vi "SaccadeAnalyser - Auto Select Channels.vi"(11 "plane":T1=enum."Yaw" caption="Impulse Plane") -> (1 "Position Response Channel":u16(ring)=7 items=["Hz Position-in-Head", "Hz Velocity-in-Head", "Hy Position-in-Head", "Hy Velocity-in-Head", "Hx Position-in-Head", "Hx Velocity-in-Head", "Hl Velocity-in-Head", "Hr Velocity-in-Head", "Lx Position-in-Head", "Ly Position-in-Head", "Lz Position-in-Head", "Lx Velocity-in-Head", "Ly Velocity-in-Head", "Lz Velocity-in-Head", "Ll Velocity-in-Head", "Lr Velocity-in-Head", "Rx Position-in-Head", "Ry Position-in-Head", "Rz Position-in-Head", "Rx Velocity-in-Head", "Ry Velocity-in-Head", "Rz Velocity-in-Head", "Rl Velocity-in-Head", "Rr Velocity-in-Head", "Target on/off", "aux input 1", "aux input 2", " ", "", "", "", "Target Hor", "Target Ver", ""], 2 "Velocity Response Channel":u16(ring)=7 items=["Hz Position-in-Head", "Hz Velocity-in-Head", "Hy Position-in-Head", "Hy Velocity-in-Head", "Hx Position-in-Head", "Hx Velocity-in-Head", "Hl Velocity-in-Head", "Hr Velocity-in-Head", "Lx Position-in-Head", "Ly Position-in-Head", "Lz Position-in-Head", "Lx Velocity-in-Head", "Ly Velocity-in-Head", "Lz Velocity-in-Head", "Ll Velocity-in-Head", "Lr Velocity-in-Head", "Rx Position-in-Head", "Ry Position-in-Head", "Rz Position-in-Head", "Rx Velocity-in-Head", "Ry Velocity-in-Head", "Rz Velocity-in-Head", "Rl Velocity-in-Head", "Rr Velocity-in-Head", "Target on/off", "aux input 1", "aux input 2", " ", "", "", "", "Target Hor", "Target Ver", ""], 3 "Stimulus Channel":u16(ring)=7 items=["Hz Position-in-Head", "Hz Velocity-in-Head", "Hy Position-in-Head", "Hy Velocity-in-Head", "Hx Position-in-Head", "Hx Velocity-in-Head", "Hl Velocity-in-Head", "Hr Velocity-in-Head", "Lx Position-in-Head", "Ly Position-in-Head", "Lz Position-in-Head", "Lx Velocity-in-Head", "Ly Velocity-in-Head", "Lz Velocity-in-Head", "Ll Velocity-in-Head", "Lr Velocity-in-Head", "Rx Position-in-Head", "Ry Position-in-Head", "Rz Position-in-Head", "Rx Velocity-in-Head", "Ry Velocity-in-Head", "Rz Velocity-in-Head", "Rl Velocity-in-Head", "Rr Velocity-in-Head", "Target on/off", "aux input 1", "aux input 2", " ", "", "", "", "Target Hor", "Target Ver", ""])   [LabVIEW 2016]
uses:
  Type Definitions/Saccade Analyser Impulse Plane.ctl
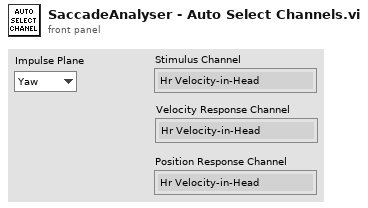
[diagram p1: front panel]
types:
  T1 = typedef "Saccade Analyser Impulse Plane.ctl" = enum16{"Other", "Yaw", "Pitch", "Roll", "LARP", "RALP"}
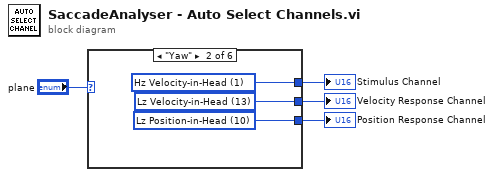
[diagram p0: block diagram]
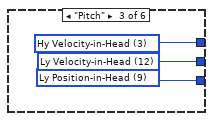
[diagram p3: hidden frame]
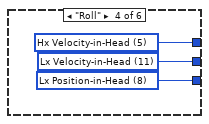
[diagram p4: hidden frame]
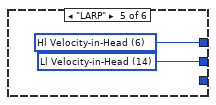
[diagram p5: hidden frame]
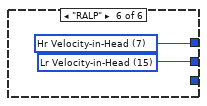
[diagram p6: hidden frame]
diagram:
  n1 = case shown="\"Yaw\"" "plane" {
    tunnel: [_ w7 w10 w13 w15 w17] -> w3
    tunnel: [_ w6 w9 w12 w14 w16] -> w2
    tunnel: [_ w5 w8 w11 _ _] -> w1
    frame "Other", Default {
      # "No default selections for these planes."
    }
    frame "Yaw" {
      w5 = u16 10 items=["Hz Position-in-Head", "Hz Velocity-in-Head", "Hy Position-in-Head", "Hy Velocity-in-Head", "Hx Position-in-Head", "Hx Velocity-in-Head", "Hl Velocity-in-Head", "Hr Velocity-in-Head", "Lx Position-in-Head", "Ly Position-in-Head", "Lz Position-in-Head", "Lx Velocity-in-Head", "Ly Velocity-in-Head", "Lz Velocity-in-Head", "Ll Velocity-in-Head", "Lr Velocity-in-Head", "Rx Position-in-Head", "Ry Position-in-Head", "Rz Position-in-Head", "Rx Velocity-in-Head", "Ry Velocity-in-Head", "Rz Velocity-in-Head", "Rl Velocity-in-Head", "Rr Velocity-in-Head", "Target on/off", "aux input 1", "aux input 2", " ", "", "", "", "Target Hor", "Target Ver", ""] ("ring_response channel")
      w6 = u16 13 items=["Hz Position-in-Head", "Hz Velocity-in-Head", "Hy Position-in-Head", "Hy Velocity-in-Head", "Hx Position-in-Head", "Hx Velocity-in-Head", "Hl Velocity-in-Head", "Hr Velocity-in-Head", "Lx Position-in-Head", "Ly Position-in-Head", "Lz Position-in-Head", "Lx Velocity-in-Head", "Ly Velocity-in-Head", "Lz Velocity-in-Head", "Ll Velocity-in-Head", "Lr Velocity-in-Head", "Rx Position-in-Head", "Ry Position-in-Head", "Rz Position-in-Head", "Rx Velocity-in-Head", "Ry Velocity-in-Head", "Rz Velocity-in-Head", "Rl Velocity-in-Head", "Rr Velocity-in-Head", "Target on/off", "aux input 1", "aux input 2", " ", "", "", "", "Target Hor", "Target Ver", ""] ("ring_response channel")
      w7 = u16 1 items=["Hz Position-in-Head", "Hz Velocity-in-Head", "Hy Position-in-Head", "Hy Velocity-in-Head", "Hx Position-in-Head", "Hx Velocity-in-Head", "Hl Velocity-in-Head", "Hr Velocity-in-Head", "Lx Position-in-Head", "Ly Position-in-Head", "Lz Position-in-Head", "Lx Velocity-in-Head", "Ly Velocity-in-Head", "Lz Velocity-in-Head", "Ll Velocity-in-Head", "Lr Velocity-in-Head", "Rx Position-in-Head", "Ry Position-in-Head", "Rz Position-in-Head", "Rx Velocity-in-Head", "Ry Velocity-in-Head", "Rz Velocity-in-Head", "Rl Velocity-in-Head", "Rr Velocity-in-Head", "Target on/off", "aux input 1", "aux input 2", " ", "", "", "", "Target Hor", "Target Ver", ""] ("ring_stimulus channel")
    }
    frame "Pitch" {
      w8 = u16 9 items=["Hz Position-in-Head", "Hz Velocity-in-Head", "Hy Position-in-Head", "Hy Velocity-in-Head", "Hx Position-in-Head", "Hx Velocity-in-Head", "Hl Velocity-in-Head", "Hr Velocity-in-Head", "Lx Position-in-Head", "Ly Position-in-Head", "Lz Position-in-Head", "Lx Velocity-in-Head", "Ly Velocity-in-Head", "Lz Velocity-in-Head", "Ll Velocity-in-Head", "Lr Velocity-in-Head", "Rx Position-in-Head", "Ry Position-in-Head", "Rz Position-in-Head", "Rx Velocity-in-Head", "Ry Velocity-in-Head", "Rz Velocity-in-Head", "Rl Velocity-in-Head", "Rr Velocity-in-Head", "Target on/off", "aux input 1", "aux input 2", " ", "", "", "", "Target Hor", "Target Ver", ""] ("ring_response channel")
      w9 = u16 12 items=["Hz Position-in-Head", "Hz Velocity-in-Head", "Hy Position-in-Head", "Hy Velocity-in-Head", "Hx Position-in-Head", "Hx Velocity-in-Head", "Hl Velocity-in-Head", "Hr Velocity-in-Head", "Lx Position-in-Head", "Ly Position-in-Head", "Lz Position-in-Head", "Lx Velocity-in-Head", "Ly Velocity-in-Head", "Lz Velocity-in-Head", "Ll Velocity-in-Head", "Lr Velocity-in-Head", "Rx Position-in-Head", "Ry Position-in-Head", "Rz Position-in-Head", "Rx Velocity-in-Head", "Ry Velocity-in-Head", "Rz Velocity-in-Head", "Rl Velocity-in-Head", "Rr Velocity-in-Head", "Target on/off", "aux input 1", "aux input 2", " ", "", "", "", "Target Hor", "Target Ver", ""] ("ring_response channel")
      w10 = u16 3 items=["Hz Position-in-Head", "Hz Velocity-in-Head", "Hy Position-in-Head", "Hy Velocity-in-Head", "Hx Position-in-Head", "Hx Velocity-in-Head", "Hl Velocity-in-Head", "Hr Velocity-in-Head", "Lx Position-in-Head", "Ly Position-in-Head", "Lz Position-in-Head", "Lx Velocity-in-Head", "Ly Velocity-in-Head", "Lz Velocity-in-Head", "Ll Velocity-in-Head", "Lr Velocity-in-Head", "Rx Position-in-Head", "Ry Position-in-Head", "Rz Position-in-Head", "Rx Velocity-in-Head", "Ry Velocity-in-Head", "Rz Velocity-in-Head", "Rl Velocity-in-Head", "Rr Velocity-in-Head", "Target on/off", "aux input 1", "aux input 2", " ", "", "", "", "Target Hor", "Target Ver", ""] ("ring_stimulus channel")
    }
    frame "Roll" {
      w11 = u16 8 items=["Hz Position-in-Head", "Hz Velocity-in-Head", "Hy Position-in-Head", "Hy Velocity-in-Head", "Hx Position-in-Head", "Hx Velocity-in-Head", "Hl Velocity-in-Head", "Hr Velocity-in-Head", "Lx Position-in-Head", "Ly Position-in-Head", "Lz Position-in-Head", "Lx Velocity-in-Head", "Ly Velocity-in-Head", "Lz Velocity-in-Head", "Ll Velocity-in-Head", "Lr Velocity-in-Head", "Rx Position-in-Head", "Ry Position-in-Head", "Rz Position-in-Head", "Rx Velocity-in-Head", "Ry Velocity-in-Head", "Rz Velocity-in-Head", "Rl Velocity-in-Head", "Rr Velocity-in-Head", "Target on/off", "aux input 1", "aux input 2", " ", "", "", "", "Target Hor", "Target Ver", ""] ("ring_response channel")
      w12 = u16 11 items=["Hz Position-in-Head", "Hz Velocity-in-Head", "Hy Position-in-Head", "Hy Velocity-in-Head", "Hx Position-in-Head", "Hx Velocity-in-Head", "Hl Velocity-in-Head", "Hr Velocity-in-Head", "Lx Position-in-Head", "Ly Position-in-Head", "Lz Position-in-Head", "Lx Velocity-in-Head", "Ly Velocity-in-Head", "Lz Velocity-in-Head", "Ll Velocity-in-Head", "Lr Velocity-in-Head", "Rx Position-in-Head", "Ry Position-in-Head", "Rz Position-in-Head", "Rx Velocity-in-Head", "Ry Velocity-in-Head", "Rz Velocity-in-Head", "Rl Velocity-in-Head", "Rr Velocity-in-Head", "Target on/off", "aux input 1", "aux input 2", " ", "", "", "", "Target Hor", "Target Ver", ""] ("ring_response channel")
      w13 = u16 5 items=["Hz Position-in-Head", "Hz Velocity-in-Head", "Hy Position-in-Head", "Hy Velocity-in-Head", "Hx Position-in-Head", "Hx Velocity-in-Head", "Hl Velocity-in-Head", "Hr Velocity-in-Head", "Lx Position-in-Head", "Ly Position-in-Head", "Lz Position-in-Head", "Lx Velocity-in-Head", "Ly Velocity-in-Head", "Lz Velocity-in-Head", "Ll Velocity-in-Head", "Lr Velocity-in-Head", "Rx Position-in-Head", "Ry Position-in-Head", "Rz Position-in-Head", "Rx Velocity-in-Head", "Ry Velocity-in-Head", "Rz Velocity-in-Head", "Rl Velocity-in-Head", "Rr Velocity-in-Head", "Target on/off", "aux input 1", "aux input 2", " ", "", "", "", "Target Hor", "Target Ver", ""] ("ring_stimulus channel")
    }
    frame "LARP" {
      w14 = u16 14 items=["Hz Position-in-Head", "Hz Velocity-in-Head", "Hy Position-in-Head", "Hy Velocity-in-Head", "Hx Position-in-Head", "Hx Velocity-in-Head", "Hl Velocity-in-Head", "Hr Velocity-in-Head", "Lx Position-in-Head", "Ly Position-in-Head", "Lz Position-in-Head", "Lx Velocity-in-Head", "Ly Velocity-in-Head", "Lz Velocity-in-Head", "Ll Velocity-in-Head", "Lr Velocity-in-Head", "Rx Position-in-Head", "Ry Position-in-Head", "Rz Position-in-Head", "Rx Velocity-in-Head", "Ry Velocity-in-Head", "Rz Velocity-in-Head", "Rl Velocity-in-Head", "Rr Velocity-in-Head", "Target on/off", "aux input 1", "aux input 2", " ", "", "", "", "Target Hor", "Target Ver", ""] ("ring_response channel")
      w15 = u16 6 items=["Hz Position-in-Head", "Hz Velocity-in-Head", "Hy Position-in-Head", "Hy Velocity-in-Head", "Hx Position-in-Head", "Hx Velocity-in-Head", "Hl Velocity-in-Head", "Hr Velocity-in-Head", "Lx Position-in-Head", "Ly Position-in-Head", "Lz Position-in-Head", "Lx Velocity-in-Head", "Ly Velocity-in-Head", "Lz Velocity-in-Head", "Ll Velocity-in-Head", "Lr Velocity-in-Head", "Rx Position-in-Head", "Ry Position-in-Head", "Rz Position-in-Head", "Rx Velocity-in-Head", "Ry Velocity-in-Head", "Rz Velocity-in-Head", "Rl Velocity-in-Head", "Rr Velocity-in-Head", "Target on/off", "aux input 1", "aux input 2", " ", "", "", "", "Target Hor", "Target Ver", ""] ("ring_stimulus channel")
    }
    frame "RALP" {
      w16 = u16 15 items=["Hz Position-in-Head", "Hz Velocity-in-Head", "Hy Position-in-Head", "Hy Velocity-in-Head", "Hx Position-in-Head", "Hx Velocity-in-Head", "Hl Velocity-in-Head", "Hr Velocity-in-Head", "Lx Position-in-Head", "Ly Position-in-Head", "Lz Position-in-Head", "Lx Velocity-in-Head", "Ly Velocity-in-Head", "Lz Velocity-in-Head", "Ll Velocity-in-Head", "Lr Velocity-in-Head", "Rx Position-in-Head", "Ry Position-in-Head", "Rz Position-in-Head", "Rx Velocity-in-Head", "Ry Velocity-in-Head", "Rz Velocity-in-Head", "Rl Velocity-in-Head", "Rr Velocity-in-Head", "Target on/off", "aux input 1", "aux input 2", " ", "", "", "", "Target Hor", "Target Ver", ""] ("ring_response channel")
      w17 = u16 7 items=["Hz Position-in-Head", "Hz Velocity-in-Head", "Hy Position-in-Head", "Hy Velocity-in-Head", "Hx Position-in-Head", "Hx Velocity-in-Head", "Hl Velocity-in-Head", "Hr Velocity-in-Head", "Lx Position-in-Head", "Ly Position-in-Head", "Lz Position-in-Head", "Lx Velocity-in-Head", "Ly Velocity-in-Head", "Lz Velocity-in-Head", "Ll Velocity-in-Head", "Lr Velocity-in-Head", "Rx Position-in-Head", "Ry Position-in-Head", "Rz Position-in-Head", "Rx Velocity-in-Head", "Ry Velocity-in-Head", "Rz Velocity-in-Head", "Rl Velocity-in-Head", "Rr Velocity-in-Head", "Target on/off", "aux input 1", "aux input 2", " ", "", "", "", "Target Hor", "Target Ver", ""] ("ring_stimulus channel")
    }
  }
  "Stimulus Channel" <- w3
  "Velocity Response Channel" <- w2
  "Position Response Channel" <- w1
